vi "Motic Release Camera.vi"(8 "error in (no error)":errorcluster, 11 "camera":i32) -> (0 "error out":errorcluster)   [LabVIEW 2012, in "MoticApi.lvlib"]
doc: "MOTICAPI void Motic_ReleaseCamera(MUCam_Handle camera);"
uses:
  MoticApi.lvlib
  MoticApi.dll
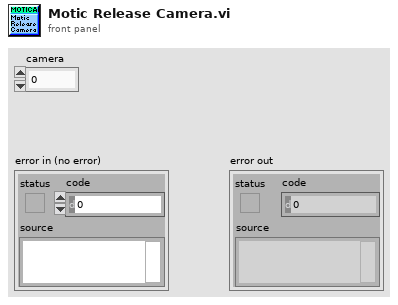
[diagram p1: front panel]
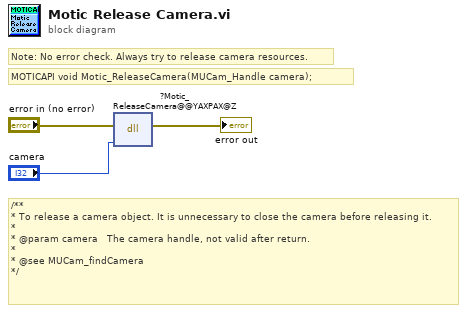
[diagram p0: block diagram]
diagram:
  # "/**\n* To release a camera object. It is unnecessary to close the camera before releasing it.\n*\n* @param camera   The camera handle, not valid after return.\n*\n* @see MUCam_findCamera\n*/"
  # "Note: No error check. Always try to release camera resources."
  # "MOTICAPI void Motic_ReleaseCamera(MUCam_Handle camera);"
  n1 = dll-call lib="C:/Users/TTS-Digital/Desktop/MoticApi/MoticApi_git/MoticApi/MoticApi.*" fn="?Motic_ReleaseCamera@@YAXPAX@Z"(error in="error in (no error)", "camera"="camera") -> (error out=→"error out":errorcluster)  [unwired: 4 in, 1 out]
